vi "Configure Multi Eval Meas Trigger Source.vi"(6 "Minimum Trigger Gap (0)":dbl format="%^.3e", 7 "Trigger Threshold (-30.00)":dbl=-30.0 format="%^.3e", 8 "error in (no error)":errorcluster, 9 "Source (\"IF Power\")":string="IF Power", 10 "Instance (1)":i32=1, 11 "VISA resource name":refnum<visa-resource-name>) -> (0 "error out":errorcluster, 3 "VISA resource name out":refnum<visa-resource-name>)   [LabVIEW 2020, in "Rohde&Schwarz CMP LR WPAN Measurement.lvlib"]
doc: "Configures multi evaluation measurement trigger subsystem.\n\nAttributes:\nRSCMPLRWM_ATTR_MULTIEVAL_TRIGGER_SOURCE\nRSCMPLRWM_ATTR_MULTIEVAL_TRIGGER_THRESHOLD\nRSCMPLRWM_ATTR_MULTIEVAL_MINIMUM_TRIGGER_GAP\n\nRemote-control commands:\nTRIGger:WPAN:MEAS<i>:MEValuation:SOURce\nTRIGger:WPAN:MEAS<i>:MEValuation:THReshold\nCONFigure:WPAN:MEAS<i>:MEValuation:TRIGger:MGAP"
uses:
  <instrlib>/Rohde&Schwarz CMP LR WPAN Measurement/Rohde&Schwarz CMP LR WPAN Measurement.lvlib
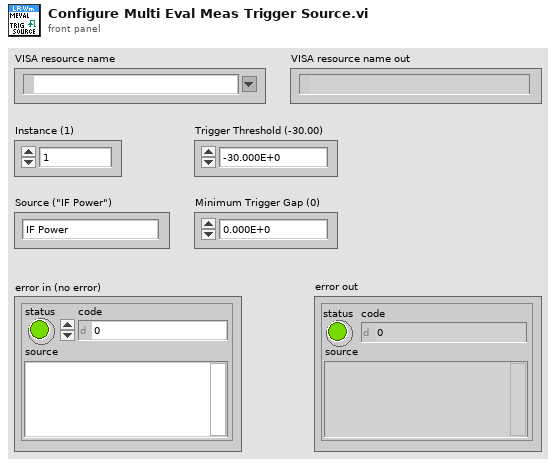
[diagram p1: front panel]
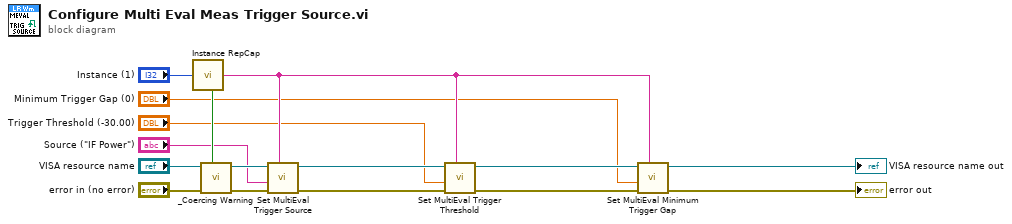
[diagram p0: block diagram]
diagram:
  n1 = call <instrlib>:"Instance RepCap.vi"("Instance In"="Instance (1)") -> ("In Range?"=w10:bool, "RepCap Identifier Out"=w9:string)  [unwired: 1 in]
  n2 = call <instrlib>:"_Coercing Warning.vi"("In Range?"=w10, "error in (no error)"="error in (no error)", "VISA resource name"="VISA resource name") -> ("error out"=w6:errorcluster, "VISA resource name out"=w5:refnum<visa-resource-name>)  [unwired: 7 in]
  n3 = call "Set MultiEval Trigger Source"("Repeated Capabilities"=w9, "error in (no error)"=w6, "MultiEval Trigger Source ()"="Source (\"IF Power\")", "instrument handle"=w5) -> ("error out"=w15:errorcluster, "instrument handle out"=w16:refnum<visa-resource-name>)  [unwired: 6 in]
  n4 = call "Set MultiEval Trigger Threshold"("Repeated Capabilities"=w9, "error in (no error)"=w15, "MultiEval Trigger Threshold (0.0)"="Trigger Threshold (-30.00)", "instrument handle"=w16) -> ("error out"=w11:errorcluster, "instrument handle out"=w12:refnum<visa-resource-name>)  [unwired: 6 in]
  n5 = call "Set MultiEval Minimum Trigger Gap"("Repeated Capabilities"=w9, "error in (no error)"=w11, "MultiEval Minimum Trigger Gap (0.0)"="Minimum Trigger Gap (0)", "instrument handle"=w12) -> ("error out"=→"error out":errorcluster, "instrument handle out"=→"VISA resource name out":refnum<visa-resource-name>)  [unwired: 6 in]
